vi "To Pretty String (Numeric).vi"(7 "enable LabVIEW extensions? (T)":bool=TRUE, 8 "error in (no error)":errorcluster, 10 "indent":i32, 11 "JSON Value in":refnum<class "JSON Value.lvclass">) -> (0 "error out":errorcluster, 3 "String":string)   [LabVIEW 2016, in "JSON Value.lvclass"]
doc: "Flattens the given JSON data to a string."
uses:
  JSON Value.lvclass
  JSON Value.lvclass/JSON Value.ctl
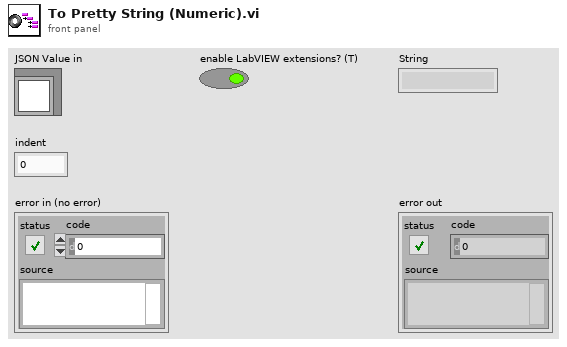
[diagram p1: front panel]
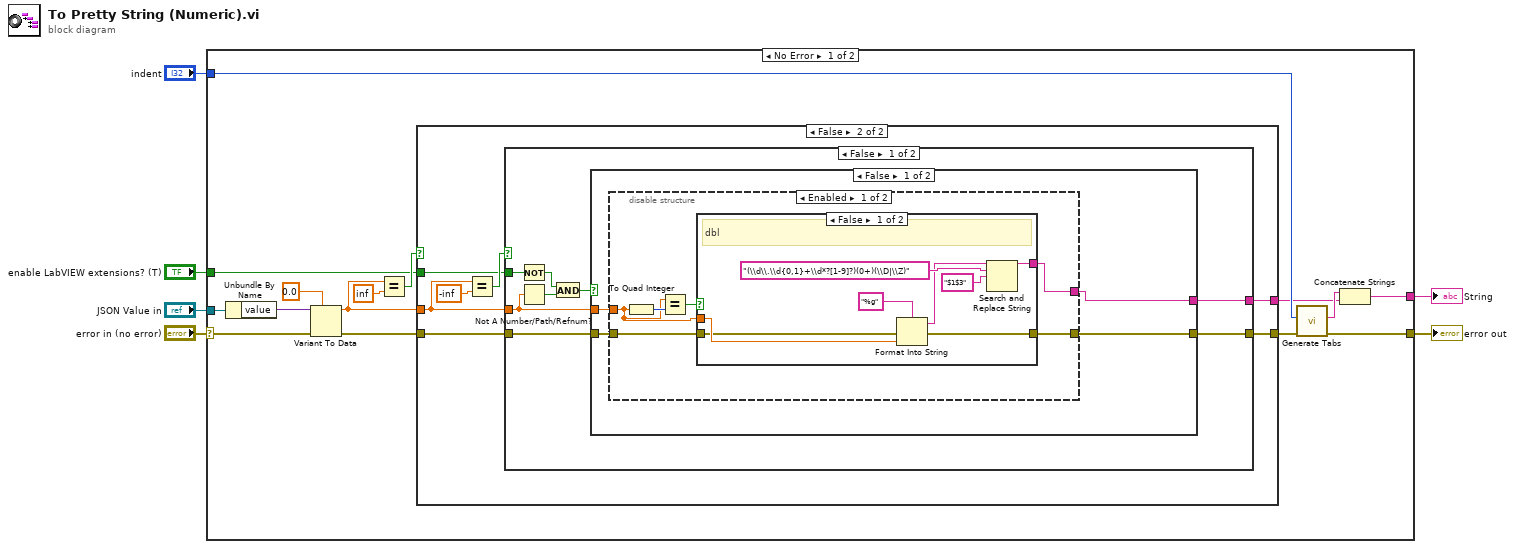
[diagram p0: block diagram]
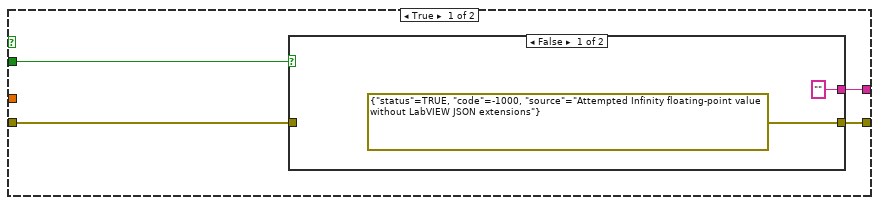
[diagram p2: hidden frame]
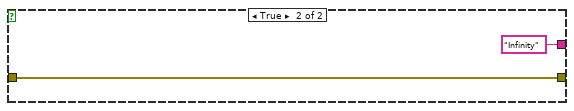
[diagram p3: hidden frame]
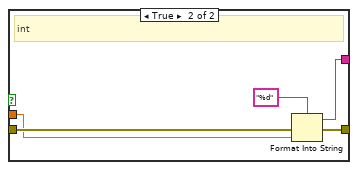
[diagram p4: hidden frame]
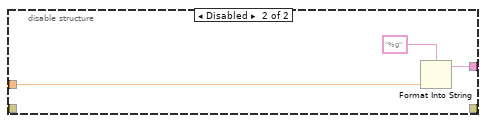
[diagram p5: hidden frame]
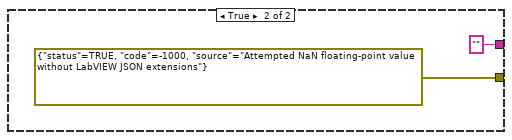
[diagram p6: hidden frame]
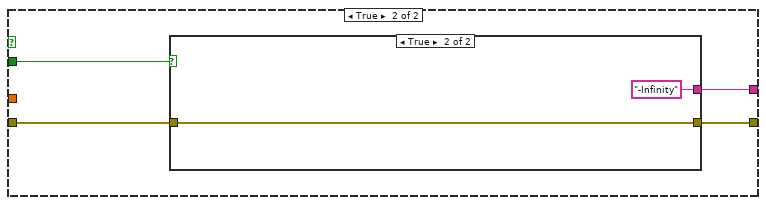
[diagram p7: hidden frame]
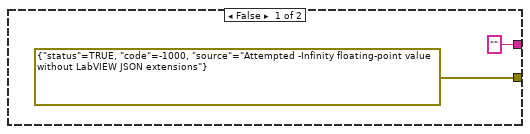
[diagram p8: hidden frame]
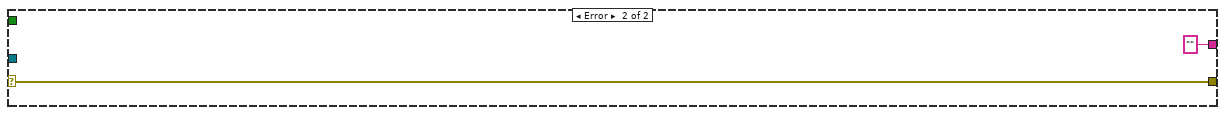
[diagram p9: hidden frame]
diagram:
  n1 = case shown="No Error" "error in (no error)" {
    selector: "error in (no error)" -> [w20 w82]
    tunnel: "JSON Value in" -> [w21 _]
    tunnel: [w8 ""] -> w4
    tunnel: [w7 w82] -> w3
    tunnel: "enable LabVIEW extensions? (T)" -> [w17 _]
    tunnel: "indent" -> [w12 _]
    frame No Error {
      n2 = Unbundle By Name(w21) -> ("value"=w15:variant)
      n3 = Variant To Data(error in=w20, type=0.0 ("y"), Variant=w15) -> (data=w14:dbl, error out=w16:errorcluster)
      n4 = Equal?(x=w14, y=inf) -> (x = y?=w18:bool)
      n5 = case shown="False" w18 {
        tunnel: w16 -> [w23 w36]
        tunnel: [w25 w35] -> w9
        tunnel: [w22 w34] -> w11
        tunnel: w14 -> [_ w32]
        tunnel: w17 -> [w24 w30]
        frame True {
          n6 = case shown="False" w24 {
            tunnel: ["" "Infinity"] -> w25
            tunnel: w23 -> [_ w28]
            tunnel: [errorcluster {"status"=TRUE, "code"=-1000, "source"="Attempted Infinity floating-point value without LabVIEW JSON extensions"} ("error IO") w28] -> w22
            frame False {
            }
            frame True {
            }
          }
        }
        frame False {
          n7 = Equal?(x=w32, y=-inf) -> (x = y?=w31:bool)
          n8 = case shown="False" w31 {
            tunnel: w36 -> [w44 w74]
            tunnel: [w43 w75] -> w35
            tunnel: [w42 w76] -> w34
            tunnel: w32 -> [w38 _]
            tunnel: w30 -> [w40 w73]
            frame False {
              n9 = Not(x=w40) -> (.not. x?=w39:bool)
              n10 = Not A Number/Path/Refnum?(number/path/refnum=w38) -> (NaN/Path/Refnum?=w37:bool)
              n11 = And(x=w39, y=w37) -> (x .and. y?=w41:bool)
              n12 = case shown="False" w41 {
                tunnel: w44 -> [w48 _]
                tunnel: [w47 ""] -> w43
                tunnel: [w46 errorcluster {"status"=TRUE, "code"=-1000, "source"="Attempted NaN floating-point value without LabVIEW JSON extensions"} ("error IO")] -> w42
                tunnel: w38 -> [w45 _]
                frame False {
                  n13 = disable-structure shown="Enabled" {
                    disable-tunnel: w48 -> [w53 _]
                    disable-tunnel: [w52 w69] -> w47
                    disable-tunnel: [w51 _] -> w46
                    disable-tunnel: w45 -> [w49 w70]
                    frame Enabled {
                      n14 = To Quad Integer(1:w49) -> (0:w50:i64)
                      n15 = Equal?(x=w49, y=w50) -> (x = y?=w54:bool)
                      n16 = case shown="False" w54 {
                        tunnel: w53 -> [w60 w65]
                        tunnel: w49 -> [w62 w63]
                        tunnel: [w55 w66] -> w52
                        tunnel: [w59 w64] -> w51
                        frame False {
                          # "dbl"
                          n17 = Format Into String(format string="%g", error in=w60, w62) -> (resulting string=w56:string, error out=w59:errorcluster)  [unwired: 1 in]
                          n18 = Search and Replace String(input string=w56, search string="(\\d\\.\\d{0,1}+\\d*?[1-9]?)(0+)(\\D|\\Z)", replace string="$1$3" ("replace string (\"\")")) -> (result string=w55:string)  [unwired: 5 in, 3 out]
                        }
                        frame True {
                          # "int"
                          n19 = Format Into String(format string="%d", error in=w65, w63) -> (resulting string=w66:string, error out=w64:errorcluster)  [unwired: 1 in]
                        }
                      }
                    }
                    frame Disabled {
                      n20 = Format Into String(format string="%g", w70) -> (resulting string=w69:string)  [unwired: 2 in, 1 out]
                    }
                  }
                }
                frame True {
                }
              }
            }
            frame True {
              n21 = case shown="True" w73 {
                tunnel: ["" "-Infinity"] -> w75
                tunnel: w74 -> [_ w79]
                tunnel: [errorcluster {"status"=TRUE, "code"=-1000, "source"="Attempted -Infinity floating-point value without LabVIEW JSON extensions"} ("error IO") w79] -> w76
                frame False {
                }
                frame True {
                }
              }
            }
          }
        }
      }
      n22 = call "Generate Tabs.vi"("error in (no error)"=w11, "indent"=w12) -> ("error out"=w7:errorcluster, "Tabs"=w10:string)  [unwired: 8 in]
      n23 = Concatenate Strings(w10, w9) -> (w8:string)
    }
    frame Error {
    }
  }
  "String" <- w4
  "error out" <- w3
